vi "Get All SLSC Switch Properties.vi"(8 "error in":errorcluster, 11 "ni-switch custom device in":T2 format="%.0x") -> (0 "error out":errorcluster, 2 "properties":T1, 3 "ni-switch custom device out":T2 format="%.0x")   [LabVIEW 2017, in "NI-SWITCH Scripting.lvlib"]
uses:
  NI-SWITCH Scripting.lvlib
  <vilib>/NI Veristand/Custom Device API/Custom Device Item Ref.ctl
  SLSC Switch All Properties.ctl
  <vilib>/NI VeriStand/Custom Device API/Custom Device API.lvlib
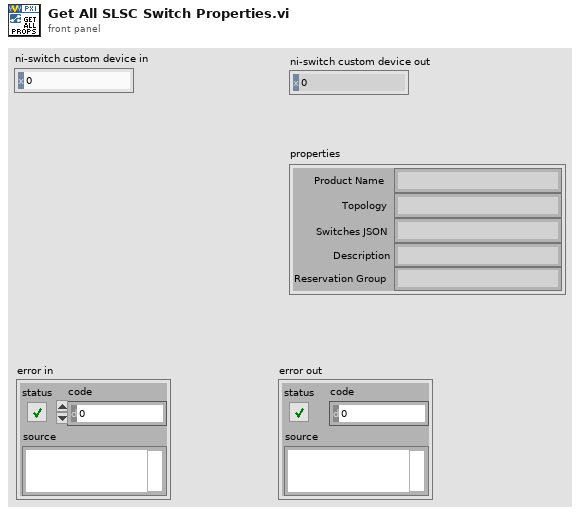
[diagram p1: front panel]
types:
  T1 = typedef "NI-SWITCH Scripting.lvlib/SLSC Switch All Properties.ctl" = cluster{"Product Name":string, "Topology":string, "Switches JSON":string, "Description":string, "Reservation Group":string}
  T2 = typedef "Custom Device API.lvlib/Custom Device Item Ref.ctl" = u64
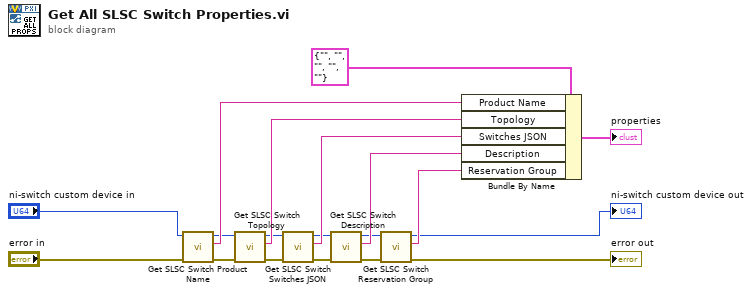
[diagram p0: block diagram]
diagram:
  n1 = call "Get SLSC Switch Product Name.vi"("error in"="error in", "slsc switch custom device in"="ni-switch custom device in") -> ("error out"=w4:errorcluster, "product name"=w15:string, "slsc switch custom device out"=w5:T2)  [unwired: 7 in]
  n2 = call "Get SLSC Switch Topology.vi"("error in"=w4, "slsc switch custom device in"=w5) -> ("error out"=w10:errorcluster, "topology"=w14:string, "slsc switch custom device out"=w11:T2)  [unwired: 7 in]
  n3 = call "Get SLSC Switch Switches JSON.vi"("error in"=w10, "slsc switch custom device in"=w11) -> ("error out"=w8:errorcluster, "switches json"=w13:string, "slsc switch custom device out"=w9:T2)  [unwired: 7 in]
  n4 = call "Get SLSC Switch Description.vi"("error in"=w8, "slsc switch custom device in"=w9) -> ("error out"=w7:errorcluster, "description"=w6:string, "slsc switch custom device out"=w2:T2)  [unwired: 7 in]
  n5 = call "Get SLSC Switch Reservation Group.vi"("error in"=w7, "slsc switch custom device in"=w2) -> ("error out"=→"error out":errorcluster, "reservation group"=w19:string, "slsc switch custom device out"=→"ni-switch custom device out":T2)  [unwired: 6 in, 1 out]
  n6 = Bundle By Name(cluster=T1 {"Product Name"="", "Topology"="", "Switches JSON"="", "Description"="", "Reservation Group"=""} ("SLSC Switch All Properties"), "Product Name"=w15, "Topology"=w14, "Switches JSON"=w13, "Description"=w6, "Reservation Group"=w19) -> (→"properties":T1)
